vi "CRYLicense Manager.vi"(11 "sAction":string) -> (2 "Cipher":string, 3 "Test Result":bool)   [LabVIEW 2013]
uses:
  CRYMainGlobal.vi
panel:
  in  "Result Listbox":i32(listbox)
  in  "buffer":u8[](array[numeric])
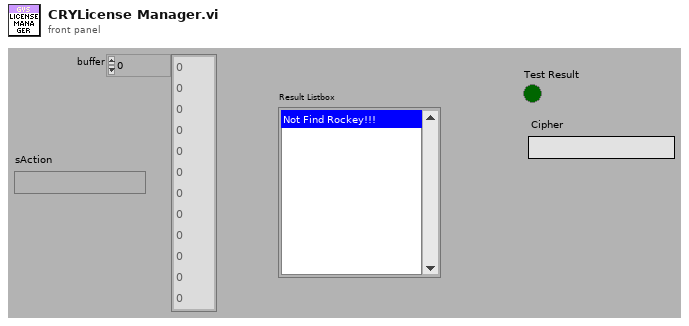
[diagram p1: front panel]
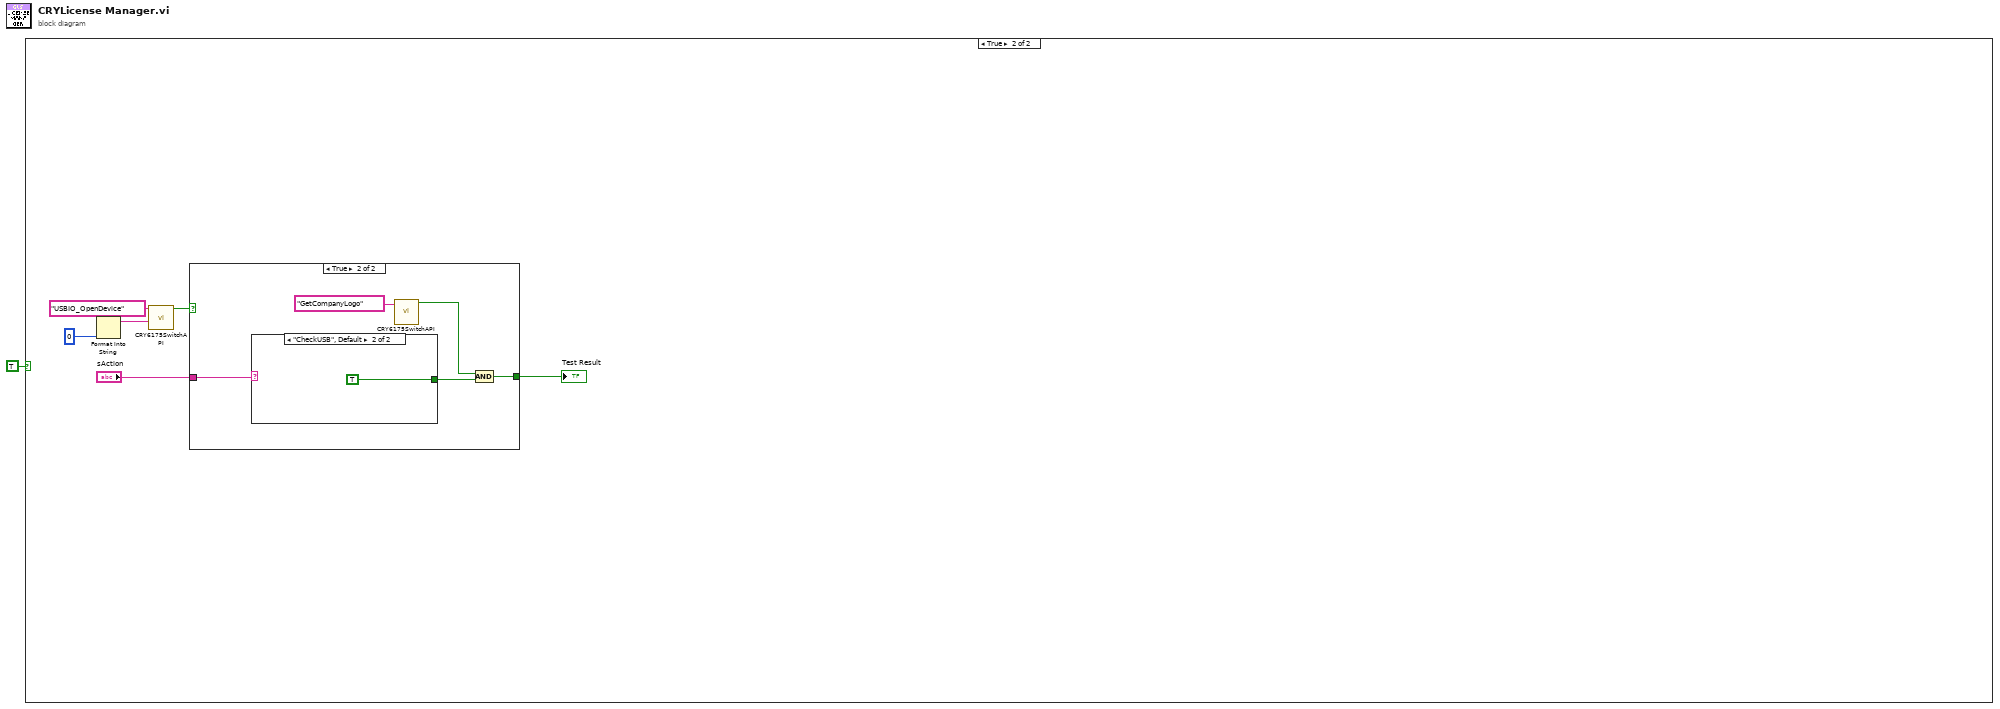
[diagram p0: block diagram]
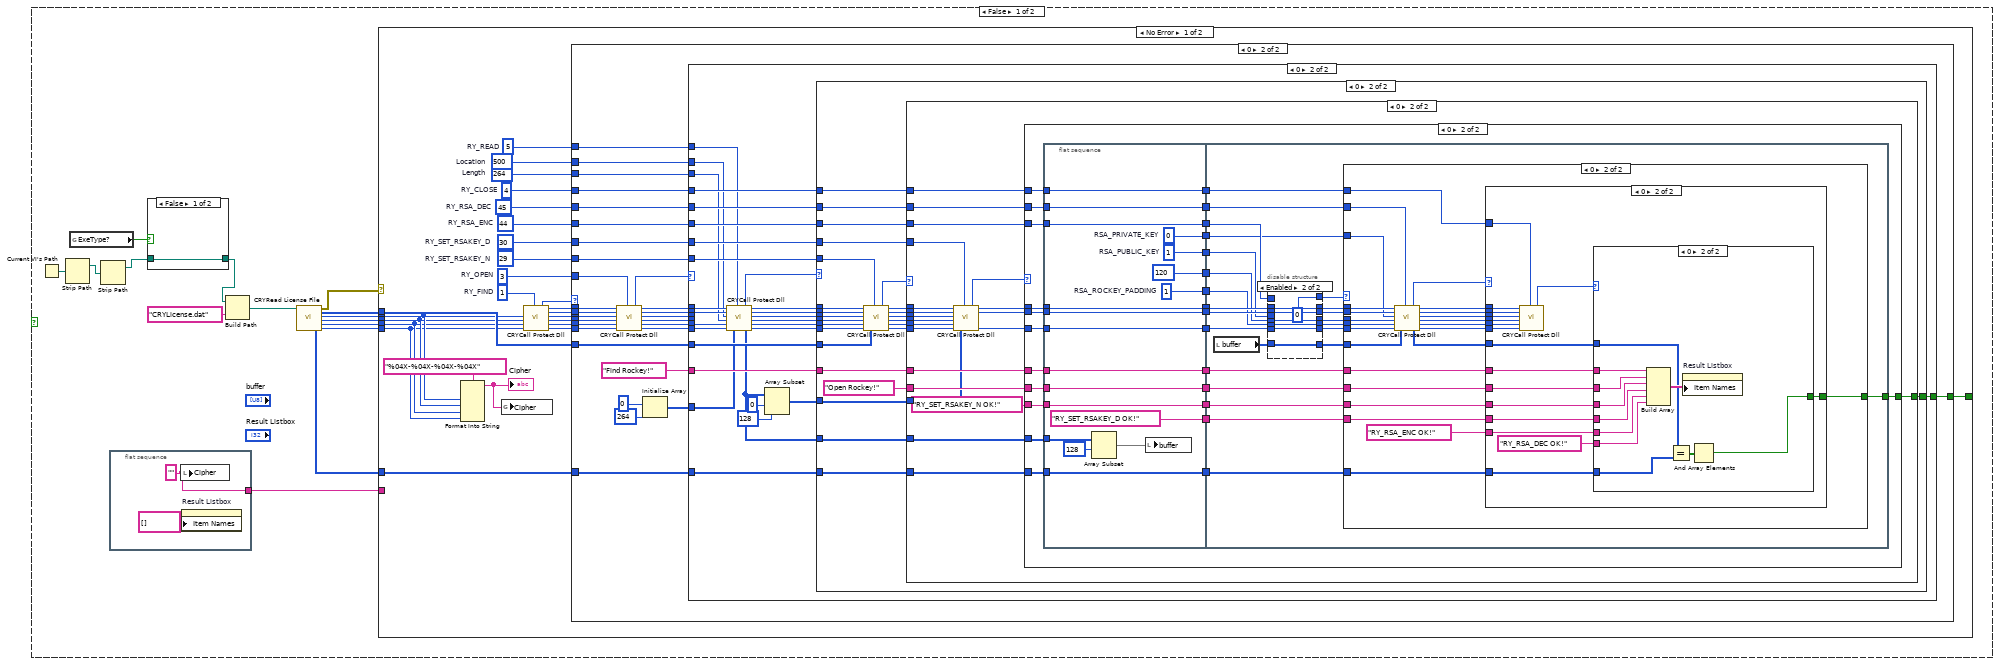
[diagram p2: hidden frame]
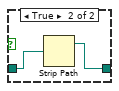
[diagram p3: hidden frame]
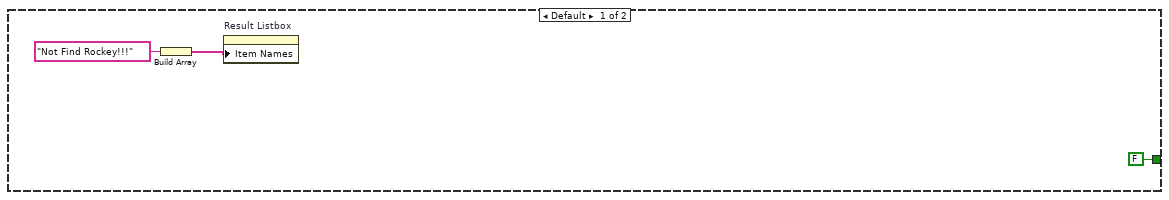
[diagram p4: hidden frame]
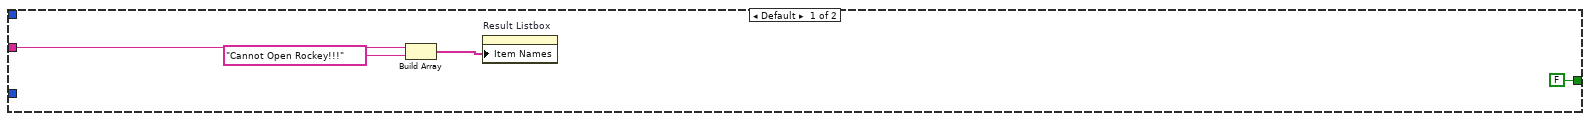
[diagram p5: hidden frame]
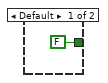
[diagram p6: hidden frame]
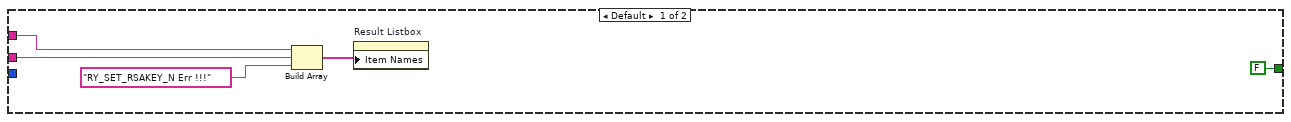
[diagram p7: hidden frame]
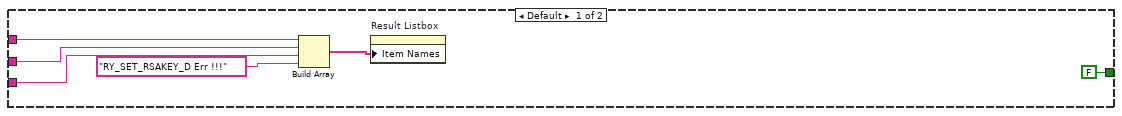
[diagram p8: hidden frame]
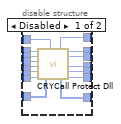
[diagram p9: hidden frame]
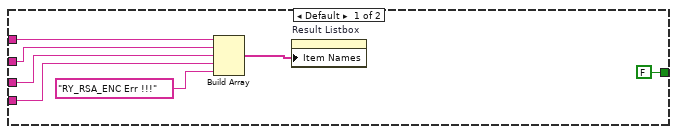
[diagram p10: hidden frame]
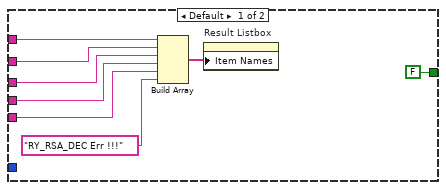
[diagram p11: hidden frame]
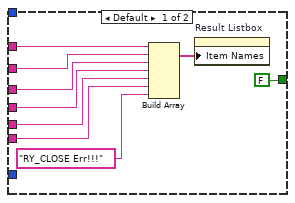
[diagram p12: hidden frame]
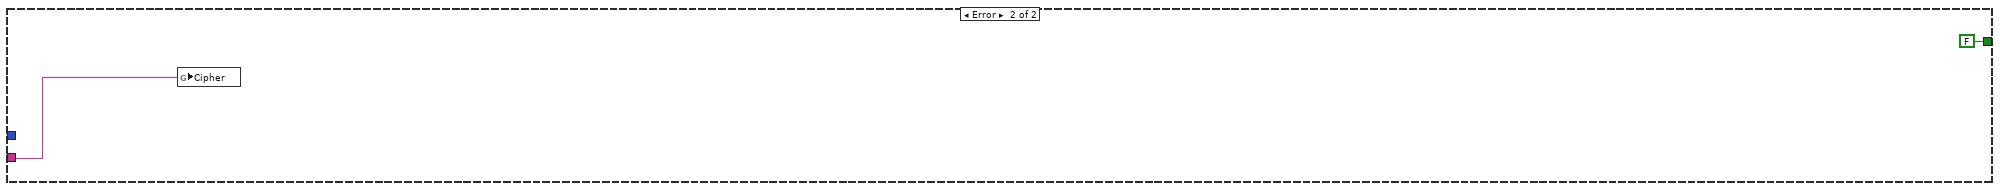
[diagram p13: hidden frame]
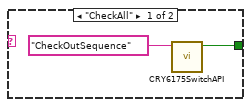
[diagram p15: hidden frame]
diagram:
  n1 = case shown="True" TRUE {
    frame False {
      n2 = Current VI's Path() -> (path=w6:path)
      n3 = Strip Path(path=w6) -> (stripped path=w5:path)  [unwired: 1 out]
      n4 = global read "CRYMainGlobal.vi" "ExeType?"() -> (w4:bool)
      n5 = Strip Path(path=w5) -> (stripped path=w3:path)  [unwired: 1 out]
      n6 = flat-sequence {
        tunnel: [w20] -> w8
        frame #0 {
          w20 = "" ("Cipher")
          n7 = local write "Cipher"(w20) -> ()
          n8 = property on="Result Listbox" class="LstBox (strict)"("Item Names"=string[] []) -> ()  [unwired: 2 in, 2 out]
        }
      }
      n9 = case shown="False" w4 {
        tunnel: w3 -> [w17 w19]
        tunnel: [w17 w18] -> w2
        frame False {
        }
        frame True {
          n10 = Strip Path(path=w19) -> (stripped path=w18:path)  [unwired: 1 out]
        }
      }
      n11 = Build Path(base path=w2, name or relative path="CRYLicense.dat") -> (appended path=w7:path)
      n12 = call "CRYRead License File.vi"("License File Name"=w7) -> ("Public Key"=w12:u8[], "License Key"=w11:u8[], "error out"=w9:errorcluster, "Data 1"=w16:u16, "Data 2"=w15:u16, "Data 3"=w14:u16, "Data 4"=w13:u16)  [unwired: 12 in]
      n13 = case shown="No Error" w9 {
        tunnel: w16 -> [w26 _]
        tunnel: w15 -> [w25 _]
        tunnel: w14 -> [w24 _]
        tunnel: w13 -> [w23 _]
        tunnel: w12 -> [w33 _]
        tunnel: w11 -> [w29 _]
        tunnel: [w28 FALSE] -> _
        tunnel: w8 -> [_ w337]
        frame No Error {
          w30 = u16 264  # Length
          w31 = u16 500  # Location
          w32 = u16 5  # RY_READ
          w34 = u16 4  # RY_CLOSE
          w35 = u16 45  # RY_RSA_DEC
          w36 = u16 44  # RY_RSA_ENC
          w37 = u16 30  # RY_SET_RSAKEY_D
          w38 = u16 29  # RY_SET_RSAKEY_N
          w45 = u16 3  # RY_OPEN
          w47 = u16 1  # RY_FIND
          n14 = Format Into String(format string="%04X-%04X-%04X-%04X", w26, w25, w24, w23) -> (resulting string=w22:string)  [unwired: 2 in, 1 out]
          "Cipher" <- w22
          n15 = global write "CRYMainGlobal.vi" "Cipher"(w22) -> ()
          n16 = call "CRYCall Protect Dll.vi"("p1"=w26, "p2"=w25, "p3"=w24, "p4"=w23, "function"=w47) -> ("return type"=w46:u16, "lp1 Out"=w42:u32, "lp2 Out"=w41:u32, "p1 Out"=w43:u16, "p2 Out"=w44:u16, "p3 Out"=w40:u16, "p4 Out"=w39:u16)  [unwired: 7 in, 1 out]
          n17 = case shown="0" w46 {
            tunnel: w45 -> [_ w79]
            tunnel: w43 -> [_ w78]
            tunnel: w44 -> [_ w77]
            tunnel: w42 -> [_ w74]
            tunnel: w41 -> [_ w73]
            tunnel: w40 -> [_ w72]
            tunnel: w39 -> [_ w71]
            tunnel: w38 -> [_ w70]
            tunnel: w37 -> [_ w63]
            tunnel: w36 -> [_ w62]
            tunnel: w35 -> [_ w61]
            tunnel: w34 -> [_ w60]
            tunnel: w33 -> [_ w59]
            tunnel: w32 -> [_ w58]
            tunnel: w31 -> [_ w54]
            tunnel: w30 -> [_ w53]
            tunnel: w29 -> [_ w52]
            tunnel: [FALSE w51] -> w28
            frame Default {
              n18 = Build Array("Not Find Rockey!!!" ("message")) -> (w49:string[])
              n19 = property on="Result Listbox" class="LstBox (strict)"("Item Names"=w49) -> ()  [unwired: 2 in, 2 out]
            }
            frame 0 {
              n20 = call "CRYCall Protect Dll.vi"("lp1"=w74, "lp2"=w73, "p1"=w78, "p2"=w77, "p3"=w72, "p4"=w71, "function"=w79) -> ("return type"=w76:u16, "lp1 Out"=w69:u32, "lp2 Out"=w68:u32, "p1 Out"=w67:u16, "p2 Out"=w66:u16, "p3 Out"=w65:u16, "p4 Out"=w64:u16)  [unwired: 5 in, 1 out]
              n21 = Initialize Array(u8 0 ("buffer"), 264 ("dimension size")) -> (w55:u8[])
              n22 = case shown="0" w76 {
                tunnel: "Find Rockey!" ("message") -> [w83 w108]
                tunnel: w70 -> [_ w111]
                tunnel: w69 -> [_ w104]
                tunnel: w68 -> [_ w103]
                tunnel: w67 -> [_ _]
                tunnel: w66 -> [_ _]
                tunnel: w65 -> [_ w102]
                tunnel: w64 -> [_ w101]
                tunnel: w63 -> [_ w110]
                tunnel: w62 -> [_ w109]
                tunnel: w61 -> [_ w107]
                tunnel: w60 -> [_ w106]
                tunnel: w59 -> [_ w105]
                tunnel: w58 -> [_ w93]
                tunnel: w55 -> [_ w92]
                tunnel: w54 -> [_ w91]
                tunnel: w53 -> [_ w90]
                tunnel: w52 -> [_ w85]
                tunnel: [FALSE w84] -> w51
                frame Default {
                  n23 = Build Array(w83, "Cannot Open Rockey!!!" ("message")) -> (w82:string[])
                  n24 = property on="Result Listbox" class="LstBox (strict)"("Item Names"=w82) -> ()  [unwired: 2 in, 2 out]
                }
                frame 0 {
                  n25 = call "CRYCall Protect Dll.vi"("lp1"=w104, "lp2"=w103, "p1"=w91, "p2"=w90, "p3"=w102, "p4"=w101, "buffer"=w92, "function"=w93) -> ("return type"=w94:u16, "buffer Out"=w86:u8[], "lp1 Out"=w100:u32, "lp2 Out"=w99:u32, "p1 Out"=w98:u16, "p2 Out"=w97:u16, "p3 Out"=w96:u16, "p4 Out"=w95:u16)  [unwired: 4 in]
                  n26 = Array Subset(array=w86, index=0, length=128) -> (w87:u8[])
                  n27 = case shown="0" w94 {
                    tunnel: w111 -> [_ w137]
                    tunnel: w100 -> [_ w136]
                    tunnel: w99 -> [_ w135]
                    tunnel: w98 -> [_ w134]
                    tunnel: w97 -> [_ w133]
                    tunnel: w96 -> [_ w132]
                    tunnel: w95 -> [_ w131]
                    tunnel: w110 -> [_ w128]
                    tunnel: w109 -> [_ w121]
                    tunnel: w108 -> [_ w120]
                    tunnel: w107 -> [_ w119]
                    tunnel: w106 -> [_ w118]
                    tunnel: w105 -> [_ w117]
                    tunnel: w87 -> [_ w116]
                    tunnel: w86 -> [_ w115]
                    tunnel: w85 -> [_ w114]
                    tunnel: [FALSE w113] -> w84
                    frame Default {
                    }
                    frame 0 {
                      n28 = call "CRYCall Protect Dll.vi"("lp1"=w136, "lp2"=w135, "p1"=w134, "p2"=w133, "p3"=w132, "p4"=w131, "buffer"=w117, "function"=w137) -> ("return type"=w130:u16, "lp1 Out"=w127:u32, "lp2 Out"=w126:u32, "p1 Out"=w125:u16, "p2 Out"=w124:u16, "p3 Out"=w123:u16, "p4 Out"=w122:u16)  [unwired: 4 in, 1 out]
                      n29 = case shown="0" w130 {
                        tunnel: "Open Rockey!" ("message") -> [w141 w149]
                        tunnel: w128 -> [_ w163]
                        tunnel: w127 -> [_ w162]
                        tunnel: w126 -> [_ w161]
                        tunnel: w125 -> [_ w160]
                        tunnel: w124 -> [_ w159]
                        tunnel: w123 -> [_ w158]
                        tunnel: w122 -> [_ w157]
                        tunnel: w121 -> [_ w151]
                        tunnel: w120 -> [w142 w150]
                        tunnel: w119 -> [_ w148]
                        tunnel: w118 -> [_ w147]
                        tunnel: w116 -> [_ w146]
                        tunnel: w115 -> [_ w145]
                        tunnel: w114 -> [_ w144]
                        tunnel: [FALSE w143] -> w113
                        frame Default {
                          n30 = Build Array(w142, w141, "RY_SET_RSAKEY_N Err !!!" ("message")) -> (w140:string[])
                          n31 = property on="Result Listbox" class="LstBox (strict)"("Item Names"=w140) -> ()  [unwired: 2 in, 2 out]
                        }
                        frame 0 {
                          n32 = call "CRYCall Protect Dll.vi"("lp1"=w162, "lp2"=w161, "p1"=w160, "p2"=w159, "p3"=w158, "p4"=w157, "buffer"=w146, "function"=w163) -> ("return type"=w156:u16, "lp1 Out"=w154:u32, "lp2 Out"=w153:u32, "p4 Out"=w152:u16)  [unwired: 4 in, 4 out]
                          n33 = case shown="0" w156 {
                            tunnel: "RY_SET_RSAKEY_N OK!" ("message") -> [w167 w179]
                            tunnel: w154 -> [_ w195]
                            tunnel: w153 -> [_ w193]
                            tunnel: w152 -> [_ w191]
                            tunnel: w151 -> [_ w190]
                            tunnel: w150 -> [w169 w183]
                            tunnel: w149 -> [w168 w181]
                            tunnel: w148 -> [_ w177]
                            tunnel: w147 -> [_ w174]
                            tunnel: w145 -> [_ w172]
                            tunnel: w144 -> [_ w171]
                            tunnel: [FALSE w170] -> w143
                            frame Default {
                              n34 = Build Array(w169, w168, w167, "RY_SET_RSAKEY_D Err !!!" ("message")) -> (w166:string[])
                              n35 = property on="Result Listbox" class="LstBox (strict)"("Item Names"=w166) -> ()  [unwired: 2 in, 2 out]
                            }
                            frame 0 {
                              n36 = flat-sequence {
                                tunnel: [w214] -> w196
                                tunnel: w195 -> [w214]
                                tunnel: [w213] -> w194
                                tunnel: w193 -> [w213]
                                tunnel: [w212] -> w192
                                tunnel: w191 -> [w212]
                                tunnel: w190 -> [w211]
                                tunnel: [w211] -> w189
                                tunnel: [w210] -> w188
                                tunnel: [w209] -> w187
                                tunnel: [u16 120 ("p2")] -> w186
                                tunnel: ["RY_SET_RSAKEY_D OK!" ("message")] -> w185
                                tunnel: [w206] -> w184
                                tunnel: w183 -> [w206]
                                tunnel: [w205] -> w182
                                tunnel: w181 -> [w205]
                                tunnel: [w204] -> w180
                                tunnel: w179 -> [w204]
                                tunnel: [w203] -> w178
                                tunnel: w177 -> [w203]
                                tunnel: [w202] -> w176
                                tunnel: [w201] -> w175
                                tunnel: w174 -> [w201]
                                tunnel: [w198] -> w173
                                tunnel: w172 -> [w200]
                                tunnel: w171 -> [w198]
                                tunnel: w196 -> [w237]
                                tunnel: w194 -> [w236]
                                tunnel: w192 -> [w235]
                                tunnel: w189 -> [w234]
                                tunnel: w188 -> [w233]
                                tunnel: w187 -> [w217]
                                tunnel: w186 -> [w232]
                                tunnel: w185 -> [w227]
                                tunnel: w184 -> [w230]
                                tunnel: w182 -> [w229]
                                tunnel: w180 -> [w228]
                                tunnel: w178 -> [w226]
                                tunnel: w176 -> [w223]
                                tunnel: w175 -> [w219]
                                tunnel: w173 -> [w216]
                                tunnel: [w215] -> w170
                                frame #0 {
                                w202 = u16 0  # RSA_PRIVATE_KEY
                                w209 = u16 1  # RSA_PUBLIC_KEY
                                w210 = u16 1  # RSA_ROCKEY_PADDING
                                n37 = Array Subset(array=w200, index=128) -> (w197:u8[])  [unwired: 1 in]
                                n38 = local write "buffer"(w197) -> ()
                                }
                                frame #1 {
                                n39 = local read "buffer"() -> (w238:u8[])
                                n40 = disable-structure shown="Enabled" {
                                disable-tunnel: w238 -> [w253 w259]
                                disable-tunnel: w237 -> [w252 w258]
                                disable-tunnel: w236 -> [w251 w257]
                                disable-tunnel: w235 -> [w250 w254]
                                disable-tunnel: w234 -> [w249 _]
                                disable-tunnel: w233 -> [w248 w255]
                                disable-tunnel: w232 -> [w247 w256]
                                disable-tunnel: [w246 u16 0 ("return type")] -> w231
                                disable-tunnel: [w245 w258] -> w225
                                disable-tunnel: [w244 w257] -> w224
                                disable-tunnel: [w243 w256] -> w222
                                disable-tunnel: [w242 w255] -> w221
                                disable-tunnel: [w241 w254] -> w220
                                disable-tunnel: [w240 w259] -> w218
                                disable-tunnel: w217 -> [w239 _]
                                frame Disabled {
                                n41 = call "CRYCall Protect Dll.vi"("lp1"=w252, "lp2"=w251, "p1"=w239, "p2"=w247, "p3"=w248, "p4"=w250, "buffer"=w253, "function"=w249) -> ("return type"=w246:u16, "buffer Out"=w240:u8[], "lp1 Out"=w245:u32, "lp2 Out"=w244:u32, "p2 Out"=w243:u16, "p3 Out"=w242:u16, "p4 Out"=w241:u16)  [unwired: 4 in, 1 out]
                                }
                                frame Enabled {
                                }
                                }
                                n42 = case shown="0" w231 {
                                tunnel: w218 -> [_ w286]
                                tunnel: w230 -> [w267 w284]
                                tunnel: w229 -> [w266 w283]
                                tunnel: w228 -> [w265 w282]
                                tunnel: w227 -> [w264 w281]
                                tunnel: w226 -> [_ w291]
                                tunnel: w225 -> [_ w290]
                                tunnel: w224 -> [_ w289]
                                tunnel: w223 -> [_ w272]
                                tunnel: w222 -> [_ w288]
                                tunnel: w221 -> [_ w271]
                                tunnel: w220 -> [_ w287]
                                tunnel: w219 -> [_ w279]
                                tunnel: w216 -> [_ w270]
                                tunnel: [FALSE w268] -> w215
                                frame Default {
                                n43 = Build Array(w267, w266, w265, w264, "RY_RSA_ENC Err !!!" ("message")) -> (w263:string[])
                                n44 = property on="Result Listbox" class="LstBox (strict)"("Item Names"=w263) -> ()  [unwired: 2 in, 2 out]
                                }
                                frame 0 {
                                n45 = call "CRYCall Protect Dll.vi"("lp1"=w290, "lp2"=w289, "p1"=w272, "p2"=w288, "p3"=w271, "p4"=w287, "buffer"=w286, "function"=w291) -> ("return type"=w285:u16, "buffer Out"=w269:u8[], "lp1 Out"=w278:u32, "lp2 Out"=w277:u32, "p1 Out"=w276:u16, "p2 Out"=w275:u16, "p3 Out"=w274:u16, "p4 Out"=w273:u16)  [unwired: 4 in]
                                n46 = case shown="0" w285 {
                                tunnel: w284 -> [w299 w316]
                                tunnel: w283 -> [w298 w315]
                                tunnel: w282 -> [w297 w314]
                                tunnel: w281 -> [w296 w313]
                                tunnel: "RY_RSA_ENC OK!" ("message") -> [w295 w312]
                                tunnel: w279 -> [_ w310]
                                tunnel: w278 -> [_ w309]
                                tunnel: w277 -> [_ w308]
                                tunnel: w276 -> [_ w307]
                                tunnel: w275 -> [_ w306]
                                tunnel: w274 -> [_ w305]
                                tunnel: w273 -> [_ w304]
                                tunnel: w270 -> [_ w301]
                                tunnel: w269 -> [_ w302]
                                tunnel: [FALSE w300] -> w268
                                frame Default {
                                n47 = Build Array(w299, w298, w297, w296, w295, "RY_RSA_DEC Err !!!" ("message")) -> (w293:string[])
                                n48 = property on="Result Listbox" class="LstBox (strict)"("Item Names"=w293) -> ()  [unwired: 2 in, 2 out]
                                }
                                frame 0 {
                                n49 = call "CRYCall Protect Dll.vi"("lp1"=w309, "lp2"=w308, "p1"=w307, "p2"=w306, "p3"=w305, "p4"=w304, "function"=w310) -> ("return type"=w303:u16)  [unwired: 5 in, 7 out]
                                n50 = case shown="0" w303 {
                                tunnel: w316 -> [w324 w335]
                                tunnel: w315 -> [w323 w334]
                                tunnel: w314 -> [w322 w333]
                                tunnel: w313 -> [w321 w332]
                                tunnel: w312 -> [w320 w331]
                                tunnel: "RY_RSA_DEC OK!" ("message") -> [w319 w330]
                                tunnel: w302 -> [_ w329]
                                tunnel: w301 -> [_ w328]
                                tunnel: [FALSE w326] -> w300
                                frame Default {
                                n51 = Build Array(w324, w323, w322, w321, w320, w319, "RY_CLOSE Err!!!" ("message")) -> (w325:string[])
                                n52 = property on="Result Listbox" class="LstBox (strict)"("Item Names"=w325) -> ()  [unwired: 2 in, 2 out]
                                }
                                frame 0 {
                                n53 = Build Array(w335, w334, w333, w332, w331, w330) -> (w336:string[])
                                n54 = Equal?(x=w329, y=w328) -> (x = y?=w327:bool[])
                                n55 = property on="Result Listbox" class="LstBox (strict)"("Item Names"=w336) -> ()  [unwired: 2 in, 2 out]
                                n56 = And Array Elements(Boolean array=w327) -> (logical AND=w326:bool)
                                }
                                }
                                }
                                }
                                }
                                }
                                }
                              }
                            }
                          }
                        }
                      }
                    }
                  }
                }
              }
            }
          }
        }
        frame Error {
          n57 = global write "CRYMainGlobal.vi" "Cipher"(w337) -> ()
        }
      }
    }
    frame True {
      n58 = Format Into String(0) -> (resulting string=w341:string)  [unwired: 3 in, 1 out]
      n59 = call "CRY6175SwitchAPI.vi"("Parameter"=w341, "Function Name"="USBIO_OpenDevice") -> ("bResult"=w340:bool)  [unwired: 9 in]
      n60 = case shown="True" w340 {
        selector: w340 -> [w345 _]
        tunnel: [w345 w350] -> w339
        tunnel: "sAction" -> [_ w346]
        frame False {
        }
        frame True {
          n61 = case shown="\"CheckUSB\", Default" w346 {
            tunnel: [w351 TRUE ("bResult")] -> w349
            frame "CheckAll" {
              n62 = call "CRY6175SwitchAPI.vi"("Function Name"="CheckOutSequence" ("sAction")) -> ("bResult"=w351:bool)  [unwired: 10 in]
            }
            frame "CheckUSB", Default {
            }
          }
          n63 = call "CRY6175SwitchAPI.vi"("Function Name"="GetCompanyLogo" ("sAction")) -> ("bResult"=w348:bool)  [unwired: 10 in]
          n64 = Compound Arithmetic op=AND(w348, w349) -> (w350:bool)
        }
      }
      "Test Result" <- w339
    }
  }
